vi "Panel.vi"(11 "BP Item in":refnum<class "BP Item.lvclass">) -> ()   [LabVIEW 2020, in "BP Item.lvclass"]
uses:
  BP Item.lvclass
  C:/dev/LabVIEW/lv-oopanel/OOPanel/Panel/Panel.lvclass
  Blueprint/Blueprint.lvclass
  BP Item.lvclass/BP Item.ctl
  Item/Ingredient.ctl
  Item/Item.lvclass
  lv-oopanel/OOPanel/Panel/Panel.lvclass
panel:
  in  "Remove":bool
  out "Item Name":string
  in  "Qty":i32=1 min=1 step=1
  out "Item Picture":picture
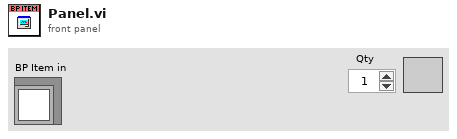
[diagram p1: front panel]
types:
  T1 = enum8{"Enabled", "Disabled", "Disabled and Grayed Out"}
  T2 = typedef "Item.lvclass/Ingredient.ctl" = cluster{"Item":refnum<class "Item.lvclass">, "Qty":dbl}
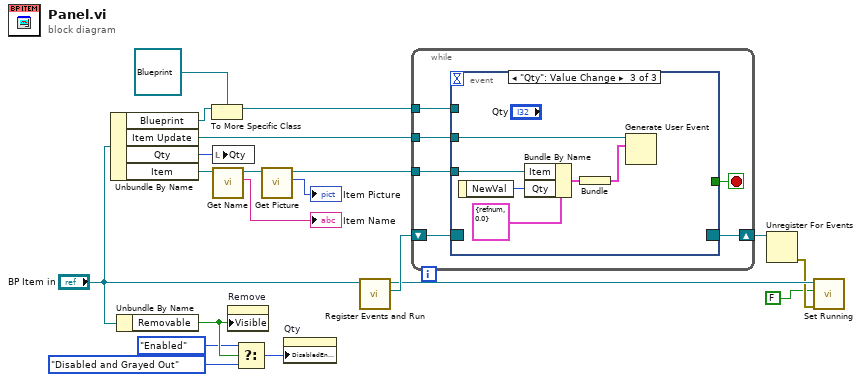
[diagram p0: block diagram]
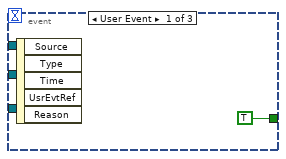
[diagram p2: hidden frame]
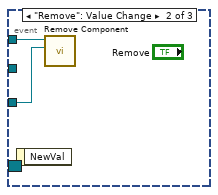
[diagram p3: hidden frame]
diagram:
  n1 = Unbundle By Name("BP Item in") -> ("Blueprint"=w20:refnum<class>, "Item Update"=w1:refnum<user-event>, "Qty"=w5:i32, "Item"=w16:refnum<class "Item.lvclass">)
  n2 = Unbundle By Name("BP Item in") -> ("Removable"=w6:bool)
  n3 = To More Specific Class(target class=refnum<class "Blueprint.lvclass"> refnum ("Blueprint.lvclass"), reference=w20) -> (specific class reference=w18:refnum<class "Blueprint.lvclass">)  [unwired: 1 in, 1 out]
  n4 = local write "Qty"(w5) -> ()
  n5 = call-dynamic "Get Name.vi"("Item in"=w16) -> ("Name"=→"Item Name":string, "Item out"=w14:refnum<class "Item.lvclass">)  [unwired: 8 in, 1 out]
  n6 = property on="Remove" class="Bool"("Visible"=w6) -> ()  [unwired: 2 in, 2 out]
  n7 = Select(t=T1."Enabled" ("Disabled"), s=w6, f=T1."Disabled and Grayed Out" ("Disabled")) -> (s? t:f=w3:T1)
  n8 = call-dynamic "Get Picture.vi"("Item in"=w14) -> ("Picture"=→"Item Picture":picture, "Item out"=w12:refnum<class "Item.lvclass">)  [unwired: 8 in, 1 out]
  n9 = property on="Qty" class="DigNum (strict)"("DisabledEnum"=w3) -> ()  [unwired: 2 in, 2 out]
  n10 = call "Register Events and Run.vi"("Panel in"="BP Item in") -> ("Panel Event Reg"=w17:refnum<event-registration>, "Panel out"=w10:refnum<class "BP Item.lvclass">)  [unwired: 8 in, 1 out]
  n11 = while {
    tunnel: w18 -> [w22]
    shift-right: [w25] -> w11
    shift-left: w17 -> [w26]
    tunnel: w12 -> [w23]
    tunnel: w1 -> [w21]
    stop <- w24 stop-if-true
    n12 = event shown="[2] \"Qty\": Value Change" {
      selector: w26 -> [_ _ _]
      dyn-events: [_ _ _] -> w25
      timeout: _ -> [_ _ _]
      tunnel: [TRUE _ _] -> w24
      tunnel: w23 -> [_ w28 w34]
      tunnel: w22 -> [_ w29 _]
      tunnel: w21 -> [_ _ w32]
      event User Event {
        n13 = event-data() -> ()  [unwired: 1 in, 5 out]
      }
      event "Remove": Value Change {
        n14 = event-data() -> ()  [unwired: 1 in, 1 out]
        n15 = call "Remove Component.vi"("Item"=w28, "Blueprint in"=w29) -> ()  [unwired: 8 in, 2 out]
      }
      event "Qty": Value Change {
        n16 = event-data() -> ("NewVal"=w33:i32)  [unwired: 1 in]
        n17 = Bundle By Name(cluster=T2 {"Item"=refnum, "Qty"=0.0} ("Ingredient"), "Item"=w34, "Qty"=w33) -> (w31:T2)
        n18 = Bundle("Ingredient"=w31) -> (w30:cluster{"Ingredient":T2})  [unwired: 1 in]
        n19 = Generate User Event(user event=w32, event data cluster=w30) -> ()  [unwired: 2 in, 2 out]
      }
    }
  }
  n20 = Unregister For Events(event registration refnum=w11) -> (error out=w9:errorcluster)  [unwired: 1 in]
  n21 = call "Set Running.vi"("error in (no error)"=w9, "Running"=FALSE, "Panel in"=w10) -> ()  [unwired: 7 in, 2 out]
